vi "GetTestInfo.vi"(11 "File selected":T2) -> (0 "Settings":T1={"Name of test"="", "Date"=timestamp(0 s since 1904-01-01), "Location"="", "Template"="", "Soundcard"="", "resolution"=32, "Sampling rate"=48000, "Ch1 Gain "=25.0, "Ch2 Gain"=10.0, "Sample time (s)"=0.3, "Pre-trigger (s)"=0.01, "Hammer Threshold"=10.0, "Positions"=12, "Taps/Position"=5, "Set Names"="", "Freq resolution"=10.0, "Hammer cutoff"=0.0, "Mic cutoff"=0.0, "Double bounce "=0.0, "Hammer Cal"=10.0, "dB Offset"=0.0, "Accel Cal"=10.0, "Vibrometer Cal"=0.0, "Mic Cal"=0.0, "Output"=2, "Voltage Cal"=0.01, "Vibrometer Port"="ASRL27::INSTR", "Range"=4, "High Pass"=2, "Bandwidth"=4, "X Range"=[{"Minimum"=200.0, "Maximum"=10000.0, "Increment"=10.0, "Minor Increment"=100.0, "Start"=200.0}, {"Minimum"=0.0, "Maximum"=0.05, "Increment"=0.025, "Minor Increment"=0.0025, "Start"=0.0}, {"Minimum"=0.0, "Maximum"=0.3, "Increment"=0.1, "Minor Increment"=0.01, "Start"=0.0}, {"Minimum"=200.0, "Maximum"=10000.0, "Increment"=10.0, "Minor Increment"=100.0, "Start"=1000.0}], "Y Range"=[{"Minimum"=-25.0, "Maximum"=0.0, "Increment"=5.0, "Minor Increment"=1.0, "Start"=-25.0}, {"Minimum"=-0.01, "Maximum"=0.1, "Increment"=0.02, "Minor Increment"=0.005, "Start"=0.0}, {"Minimum"=-0.1, "Maximum"=0.1, "Increment"=0.05, "Minor Increment"=0.01, "Start"=-0.1}, {"Minimum"=-35.0, "Maximum"=5.0, "Increment"=2.0, "Minor Increment"=0.5, "Start"=-34.0}], "dB Spread"=0.0, "Trigger"=0, "Ch_1"=25, "Ch_2"=25, "flip?"=FALSE, "60Hz"=FALSE, "Time offset"=0.0, "Piezo Cal"=0.0, "Default Notes"="", "Tom"=FALSE} {"Ch_2" min=1 step=1; "Ch_1" min=1 max=100 step=1; "Trigger" items=["Hammer (force)", "Self-tap"]; "Bandwidth" items=["1 kHz", "5 kHz", "10 kHz", "25 kHz", "50 kHz", "100 kHz"]; "High Pass" items=["Off", "13 Hz", "104 Hz"]; "Range" items=["10 mm/s", "20 mm/s", "50 mm/s", "100 mm/s", "200 mm/s", "500 mm/s", "1 m/s", "2 m/s"]; "Output" items=["Acclerometer", "Displacement", "Microphone", "Vibrometer"]; "Voltage Cal" format="%#_13g"; "Ch2 Gain" format="%#_13g"; "Ch1 Gain" format="%#_13g"; "Hammer Cal" min=0.0; "Double bounce" min=0.0; "Mic cutoff" min=0.0 format="%#_4g"; "Hammer cutoff" min=0.0 format="%#_4g"; "Freq resolution" min=0.0; "Pre-trigger (s)" format="%#_13g"; "Date" format="%<%H:%M\n%d/%m/%y>T"; "resolution" items=["16 bit"=16, "24 bit"=24, "32 bit"=32]; "Sampling rate" items=["22050 samp/s"=22050, "44100 samp/s"=44100, "48000 samp/s"=48000]}, 1 "Tags":string, 2 "Notes":string, 3 "File name":string, 4 "Instrument--Test":string, 5 "Notes Path":path, 6 "Visible?":bool, 7 "Settings Path":path)   [LabVIEW 2022 SP3]
uses:
  Curtin1_Label.ctl
  Mic/Mic_Global.vi
panel:
  out "Microphone Data":cluster{dbl, "dt":dbl, "Y":dbl[]}[](graph)
  out "Hammer Data":cluster{dbl, "dt":dbl, "Y":dbl[]}[](graph)
  # "mV/Pa"
  # "mV/m/s2"
  # "mV/mm/s"
  # "V/N"
  # "sec"
  # "sec"
  # "mV/N"
  # "Hz"
  # "a.u."
  # "dB"
  # "a.u."
  # "dB"
  # "sec"
  # "sec"
  # "sec"
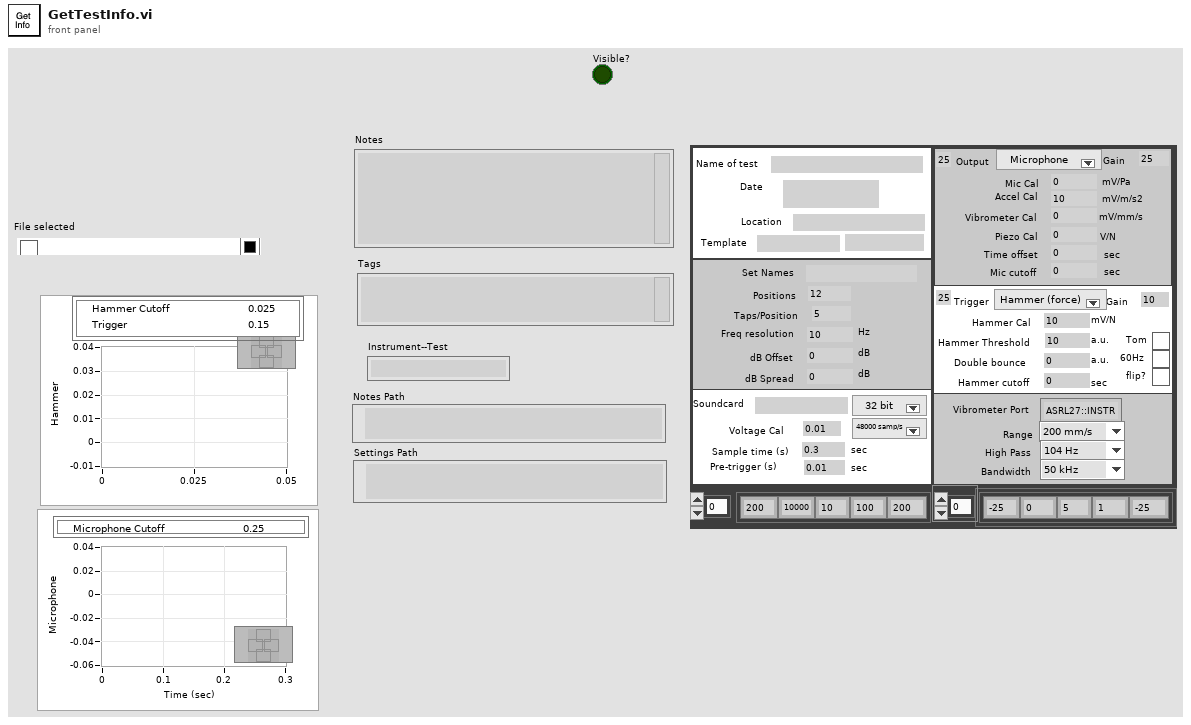
[diagram p1: front panel]
types:
  T1 = cluster{"Name of test":string, "Date":timestamp, "Location":string, "Template":string, "Soundcard":string, "resolution":u16, "Sampling rate":u16, "Ch1 Gain ":dbl, "Ch2 Gain":dbl, "Sample time (s)":dbl, "Pre-trigger (s)":dbl, "Hammer Threshold":dbl, "Positions":i16, "Taps/Position":i16, "Set Names":string, "Freq resolution":dbl, "Hammer cutoff":dbl, "Mic cutoff":dbl, "Double bounce ":dbl, "Hammer Cal":dbl, "dB Offset":dbl, "Accel Cal":dbl, "Vibrometer Cal":dbl, "Mic Cal":dbl, "Output":u16, "Voltage Cal":dbl, "Vibrometer Port":string, "Range":u16, "High Pass":u16, "Bandwidth":u16, "X Range":cluster{"Minimum":dbl, "Maximum":dbl, "Increment":dbl, "Minor Increment":dbl, "Start":dbl}[], "Y Range":cluster{"Minimum":dbl, "Maximum":dbl, "Increment":dbl, "Minor Increment":dbl, "Start":dbl}[], "dB Spread":dbl, "Trigger":u16, "Ch_1":u8, "Ch_2":u8, "flip?":bool, "60Hz":bool, "Time offset":dbl, "Piezo Cal":dbl, "Default Notes":string, "Tom":bool}
  T2 = typedef "Curtin1_Label.ctl" = cluster{"Show?":bool, "Name":string, "Color":u32, "Path":path, "Show Notes":bool}
  T3 = typedef "PreferencesControl.ctl" = cluster{"Name of test":string, "Date":timestamp, "Location":string, "Template":string, "Soundcard":string, "resolution":u16, "Sampling rate":u16, "Ch1 Gain ":dbl, "Ch2 Gain":dbl, "Sample time (s)":dbl, "Pre-trigger (s)":dbl, "Hammer Threshold":dbl, "Positions":i16, "Taps/Position":i16, "Set Names":string, "Freq resolution":dbl, "Hammer cutoff":dbl, "Mic cutoff":dbl, "Double bounce ":dbl, "Hammer Cal":dbl, "dB Offset":dbl, "Accel Cal":dbl, "Vibrometer Cal":dbl, "Mic Cal":dbl, "Output":u16, "Voltage Cal":dbl, "Vibrometer Port":refnum<visa-resource-name>, "Range":u16, "High Pass":u16, "Bandwidth":u16, "X Range":cluster{"Minimum":dbl, "Maximum":dbl, "Increment":dbl, "Minor Increment":dbl, "Start":dbl}[], "Y Range":cluster{"Minimum":dbl, "Maximum":dbl, "Increment":dbl, "Minor Increment":dbl, "Start":dbl}[], "dB Spread":dbl, "Trigger":u16, "Ch_1":u8, "Ch_2":u8, "flip?":bool, "60Hz":bool, "Time offset":dbl, "Piezo Cal":dbl, "Default Notes":string, "Tom":bool}
  T4 = cluster{"Hammer":cluster{dbl, "dt":dbl, "Y":dbl[]}[], "Microphone":cluster{dbl, "dt":dbl, "Y":dbl[]}[], "Hammer Spectrum":cluster{dbl, "dt":dbl, "Y":dbl[]}[], "FRF":cluster{dbl, "dt":dbl, "Y":dbl[]}[]}
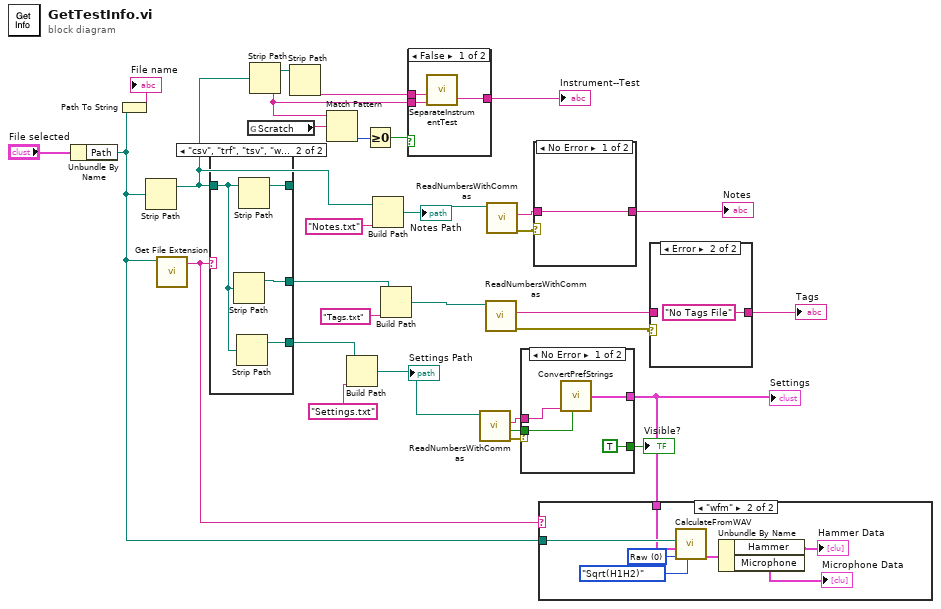
[diagram p0: block diagram]
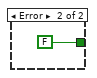
[diagram p6: hidden frame]
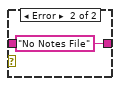
[diagram p7: hidden frame]
diagram:
  n1 = Unbundle By Name("File selected") -> ("Path"=w14:path)
  n2 = Path To String(path=w14) -> (string=→"File name":string)
  n3 = Strip Path(path=w14) -> (stripped path=w1:path)  [unwired: 1 out]
  n4 = call <vilib>:"Get File Extension.vi"("file"=w14) -> ("lowercase file extension"=w12:string)  [unwired: 6 in, 4 out]
  n5 = case shown="\"csv\", \"trf\", \"tsv\", \"wfm\"" w12 {
    tunnel: [w32 w36] -> _
    tunnel: [w32 w35] -> w28
    tunnel: w1 -> [w32 w34]
    tunnel: [w32 w33] -> w22
    frame Default {
    }
    frame "csv", "trf", "tsv", "wfm" {
      n6 = Strip Path(path=w34) -> (stripped path=w35:path)  [unwired: 1 out]
      n7 = Strip Path(path=w34) -> (stripped path=w33:path)  [unwired: 1 out]
      n8 = Strip Path(path=w34) -> (stripped path=w36:path)  [unwired: 1 out]
    }
  }
  n9 = global read "Mic_Global.vi" "Scratch"() -> (w19:string)
  n10 = Strip Path(path=w1) -> (stripped path=w24:path, name=w17:string)
  n11 = Strip Path(path=w24) -> (name=w23:string)  [unwired: 1 out]
  n12 = Match Pattern(string=w17, regular expression=w19) -> (offset past match=w18:i32)  [unwired: 1 in, 3 out]
  n13 = Build Path(base path=w22, name or relative path="Settings.txt") -> (appended path=w11:path)
  "Settings Path" <- w11
  n14 = Greater Or Equal To 0?(x=w18) -> (x >= 0?=w16:bool)
  n15 = Build Path(base path=w1, name or relative path="Notes.txt") -> (appended path=w4:path)
  "Notes Path" <- w4
  n16 = Build Path(base path=w28, name or relative path="Tags.txt") -> (appended path=w7:path)
  n17 = case shown="False" w16 {
    tunnel: [w39 w40] -> w25
    tunnel: w23 -> [w38 _]
    tunnel: w17 -> [w37 w40]
    frame False {
      n18 = call "SeparateInstrumentTest.vi"("test in"=w37, "Instrument in"=w38) -> ("Instrument -- test out"=w39:string)  [unwired: 5 in, 4 out]
    }
    frame True {
    }
  }
  "Instrument--Test" <- w25
  n19 = call "ReadNumbersWithCommas.vi"("file (use dialog)"=w11) -> ("error out"=w10:errorcluster, "comma?"=w8:bool, "text"=w9:string)  [unwired: 7 in, 1 out]
  n20 = call "ReadNumbersWithCommas.vi"("file (use dialog)"=w7) -> ("error out"=w5:errorcluster, "text"=w6:string)  [unwired: 7 in, 2 out]
  n21 = call "ReadNumbersWithCommas.vi"("file (use dialog)"=w4) -> ("error out"=w2:errorcluster, "text"=w3:string)  [unwired: 7 in, 2 out]
  n22 = case shown="No Error" w10 {
    tunnel: w9 -> [w44 _]
    tunnel: [w43 _] -> w13
    tunnel: [TRUE FALSE] -> w20
    tunnel: w8 -> [w41 _]
    frame No Error {
      n23 = call "ConvertPrefStrings.vi"("Comma?"=w41, "String In"=w44) -> ("Settings"=w43:T3)  [unwired: 8 in, 1 out]
    }
    frame Error {
    }
  }
  "Settings" <- w13
  "Visible?" <- w20
  n24 = case shown="No Error" w2 {
    tunnel: w3 -> [w46 _]
    tunnel: [w46 "No Notes File"] -> w21
    frame No Error {
    }
    frame Error {
    }
  }
  "Notes" <- w21
  n25 = case shown="\"wfm\"" w12 {
    tunnel: w14 -> [_ w54]
    tunnel: w13 -> [_ w53]
    frame Default {
    }
    frame "wfm" {
      w52 = u16 0 items=["Raw", "Volts", "Units (Pa, N, etc)"] ("View")
      n26 = call "CalculateFromWAV.vi"("Method"=enum16{"Sqrt(H1H2)", "H1", "H2"}."Sqrt(H1H2)", "View"=w52, "Settings"=w53, "path"=w54) -> ("Plots"=w50:T4)  [unwired: 3 in, 4 out]
      n27 = Unbundle By Name(w50) -> ("Hammer"=→"Hammer Data":cluster{dbl, "dt":dbl, "Y":dbl[]}[], "Microphone"=→"Microphone Data":cluster{dbl, "dt":dbl, "Y":dbl[]}[])
    }
  }
  n28 = case shown="Error" w5 {
    tunnel: w6 -> [w55 _]
    tunnel: [w55 "No Tags File"] -> w26
    frame No Error {
    }
    frame Error {
    }
  }
  "Tags" <- w26
